vi "Status Page.vi"(8 "Error in":errorcluster, 11 "INL DNL Test in":refnum<class "INL DNL Test.lvclass">) -> (0 "Error out":errorcluster, 3 "INL DNL Test out":refnum<class "INL DNL Test.lvclass">)   [LabVIEW 2020, in "INL DNL Test.lvclass"]
doc: "Status page which displays the DNL and INL results in graph. It also plots the transfer function and plot it in XY graph."
uses:
  INL DNL Test.lvclass
  D:/SDLC/Class/INL DNL Test/Test/Parent/Test.lvclass
  Typedef/User event controls.ctl
  Typedef/Queue Operation.ctl
  Class/INL DNL Test/Device/Parent/Typedef/Data Cluster.ctl
  Class/INL DNL Test/Device/Parent/Device.lvclass
  INL DNL Test.lvclass/INL DNL Test.ctl
  DNL INL Test.lvlib
panel:
  in  "Tab Control":enum32{"Status and graph", "Transfer Function"}(tab)
  out "INL Plot":cluster{"X Values":dbl[], "Y Values":dbl[]}(graph)
  out "DNL Plot":T1(graph)
  in  "Show Tranfer Function":bool
  out "INL":dbl
  out "DNL":dbl
  out "Code":i32
  out "Transfer Function":T2(graph)
  in  "Show DNL INL graph":bool
  # "Note:\nClick run test button to calculate and plot results in graph"
  # "Status and Graph"
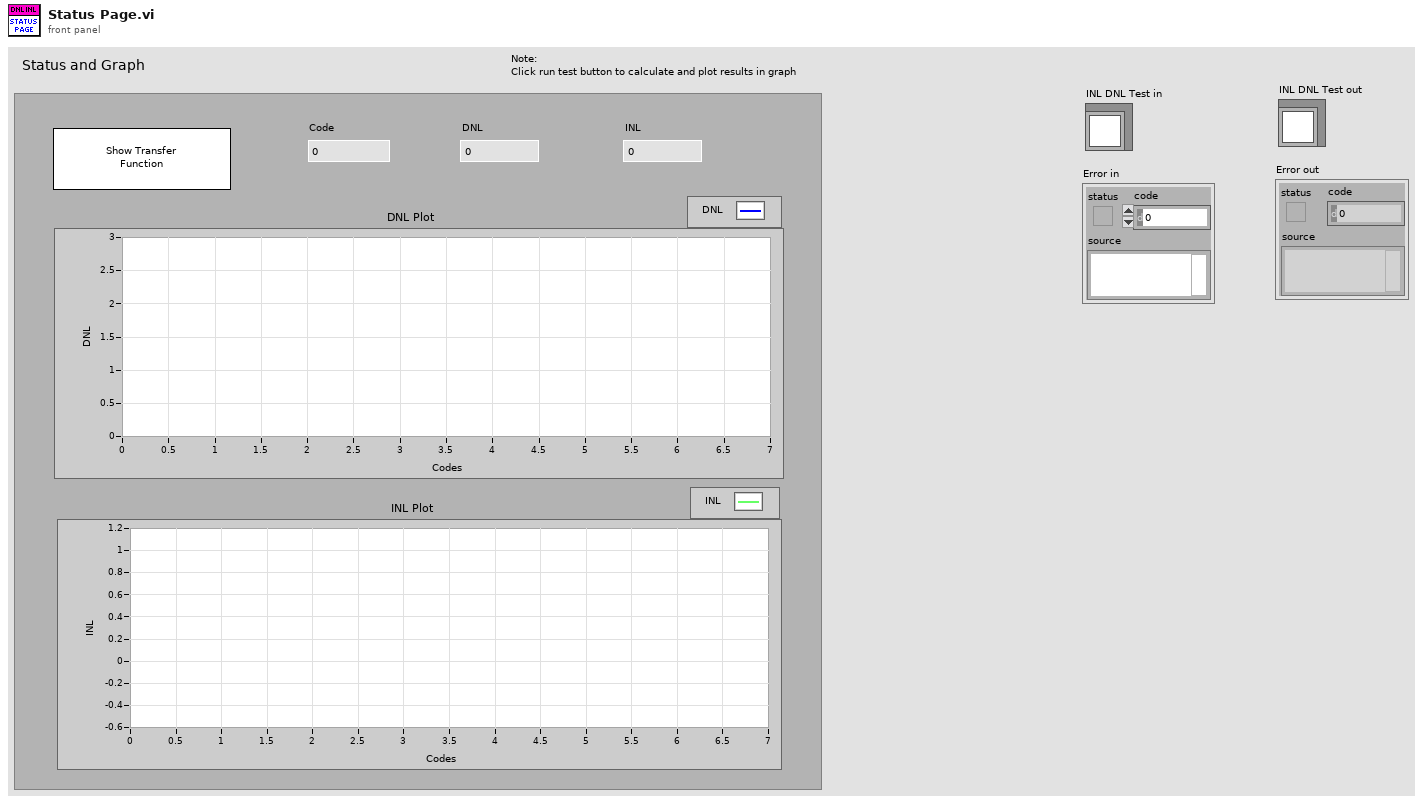
[diagram p1: front panel]
types:
  T1 = cluster{"Ideal Values":dbl[], "Deviated Values":dbl[]}
  T2 = cluster{"Ideal Vlaues":dbl[], "Deviated Values":dbl[]}[]
  T3 = typedef "DNL INL Test.lvlib/Queue Operation.ctl" = enum16{"Create Queue", "Enqueue", "Dequeue", "Enstack", "Flush Queue", "Release Queue"}
  T4 = typedef "DNL INL Test.lvlib/User event controls.ctl" = enum16{"Create", "Generate", "Run Test", "Get Ref", "Destroy"}
  T5 = typedef "Device.lvclass/Data Cluster.ctl" = cluster{"X Values":dbl[], "Y Values":dbl[]}
  T6 = typedef "LVPoint32TypeDef.ctl" = cluster{"Horizontal":i32, "Vertical":i32}
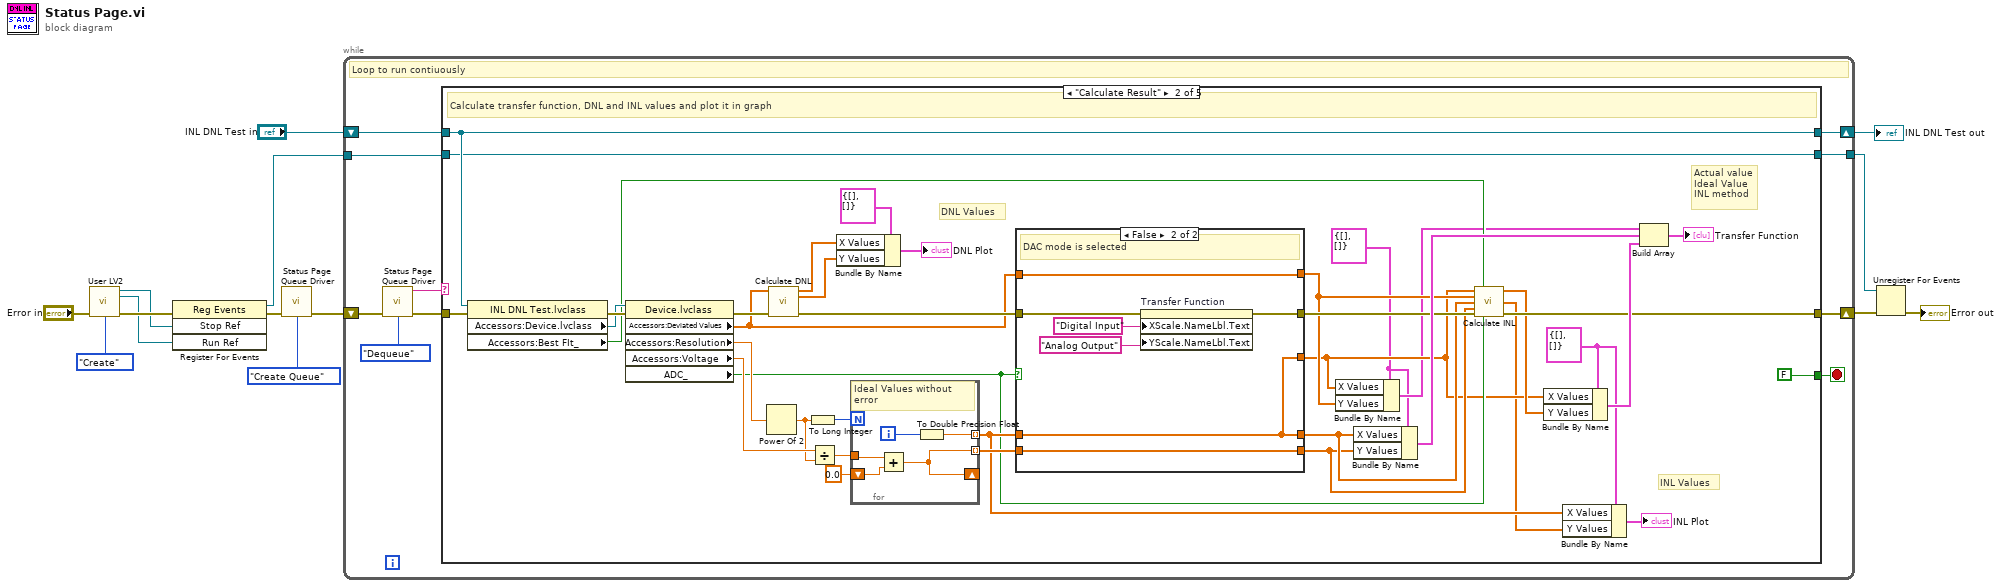
[diagram p0: block diagram]
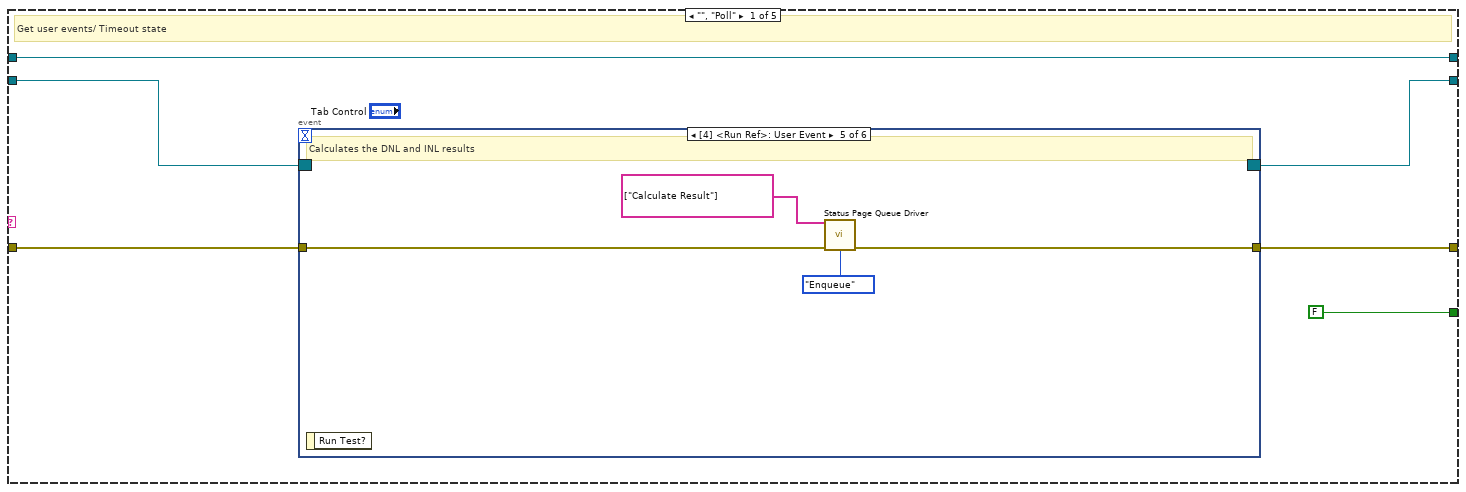
[diagram p2: hidden frame]
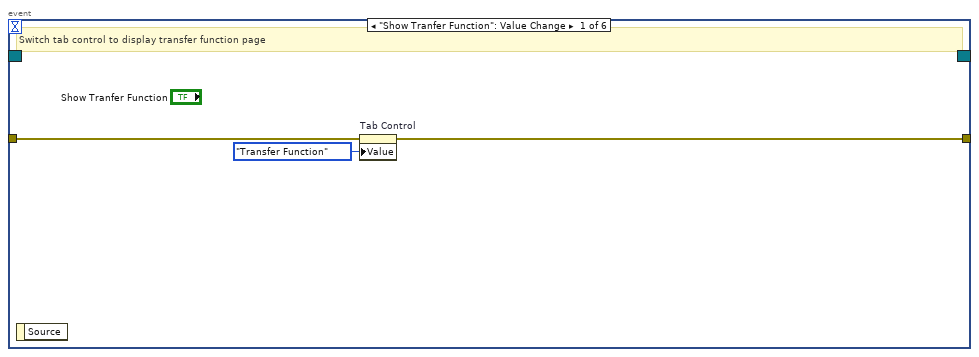
[diagram p3: hidden frame]
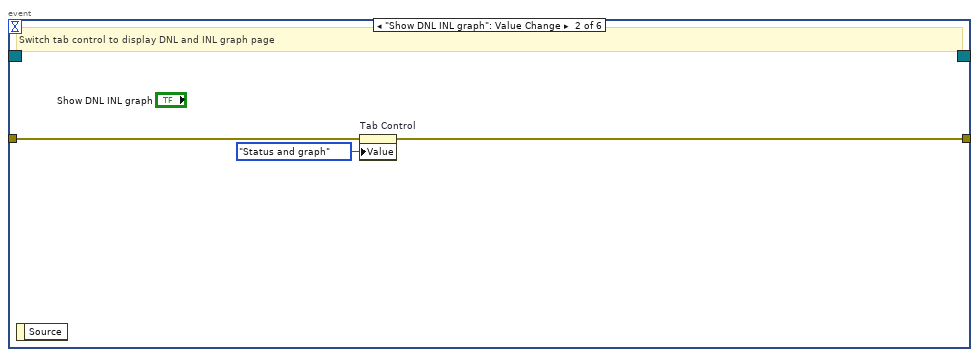
[diagram p4: hidden frame]
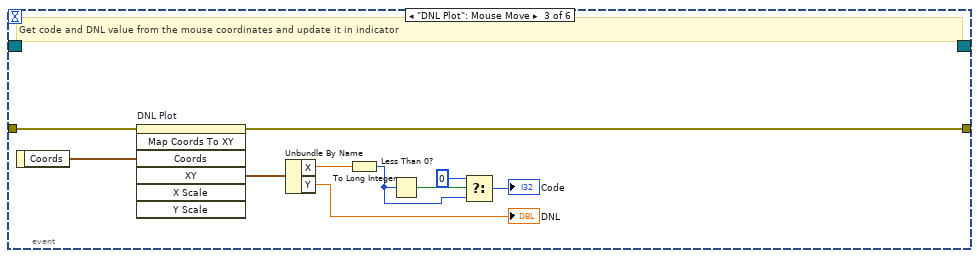
[diagram p5: hidden frame]
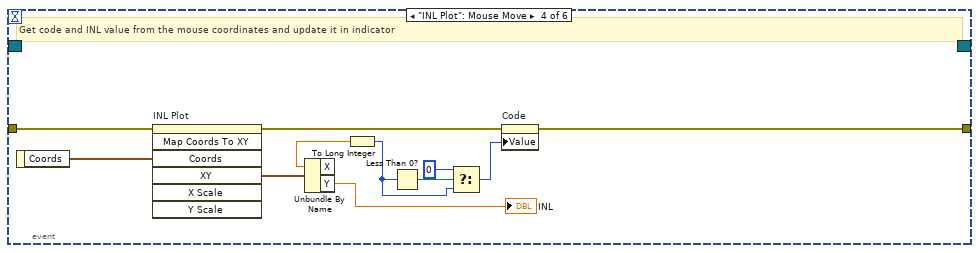
[diagram p6: hidden frame]
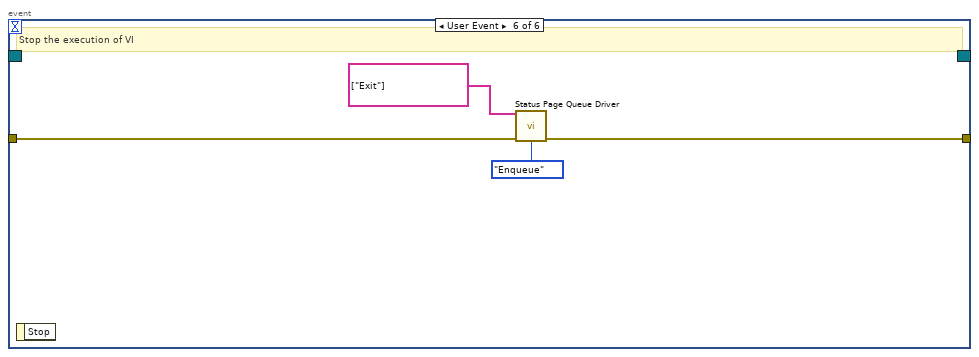
[diagram p7: hidden frame]
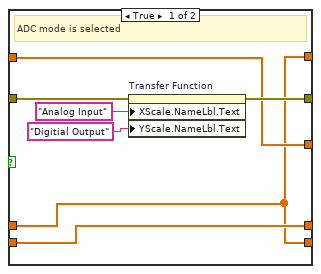
[diagram p8: hidden frame]
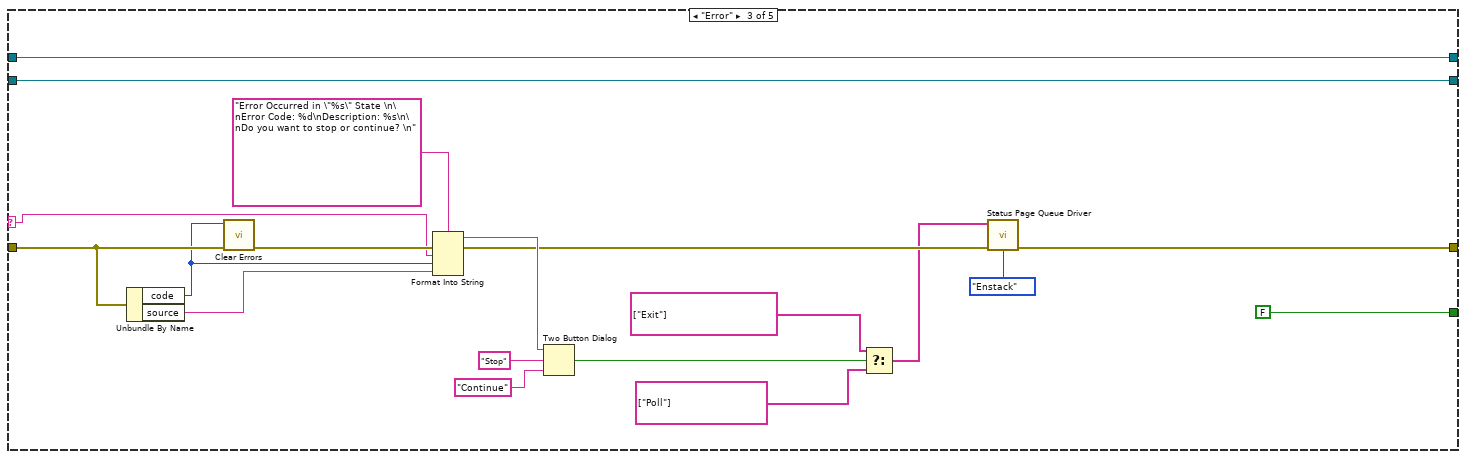
[diagram p9: hidden frame]
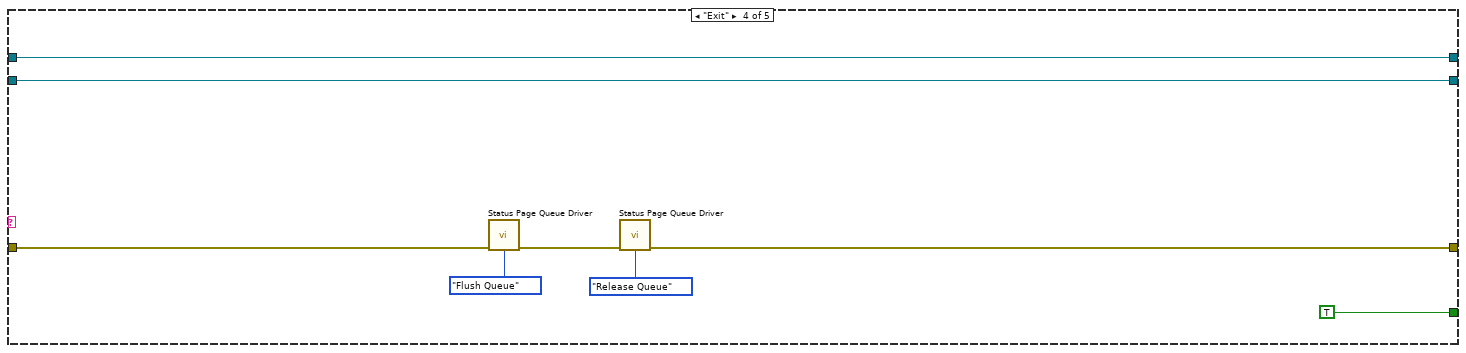
[diagram p10: hidden frame]
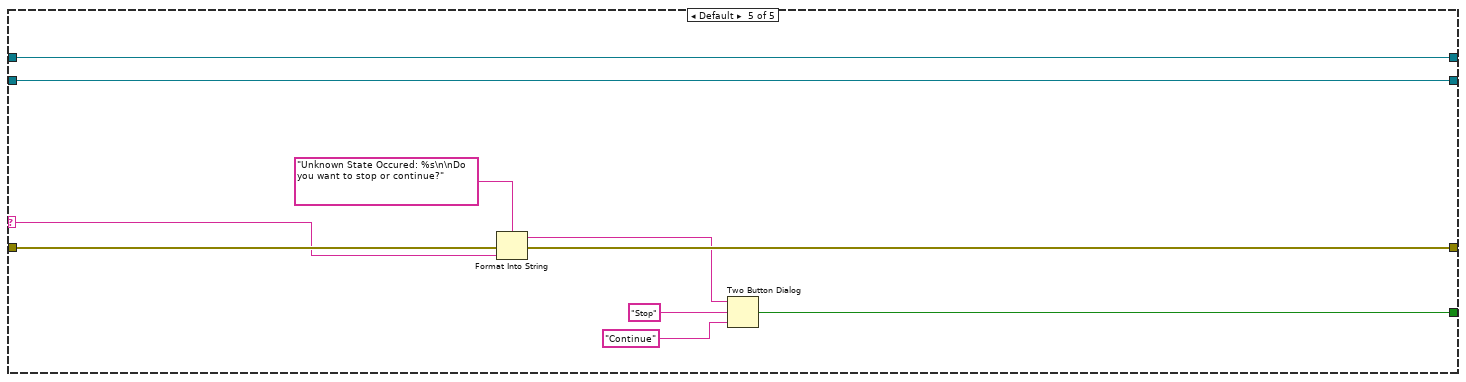
[diagram p11: hidden frame]
diagram:
  n1 = call "User LV2.vi"("Error In"="Error in", "User event controls"=User_event_controls."Create") -> ("Stop Ref"=w11:refnum<user-event>, "Run Ref"=w4:refnum<user-event>, "Error Out"=w12:errorcluster)  [unwired: 11 in]
  n2 = register-events(error in=w12, w11, w4) -> (reference out=w10:refnum<event-registration>, error out=w3:errorcluster)  [unwired: 1 in]
  n3 = call "Status Page Queue Driver.vi"("Error in"=w3, "Queue Operation"=Queue_Operation."Create Queue") -> ("Error out"=w1:errorcluster)  [unwired: 12 in, 1 out]
  n4 = while {
    shift-right: [w24] -> w9
    shift-left: w1 -> [w16]
    tunnel: w10 -> [w23]
    tunnel: [w21] -> w7
    shift-right: [w19] -> w5
    shift-left: "INL DNL Test in" -> [w20]
    stop <- w22 stop-if-true
    # "Loop to run contiuously"
    n5 = call "Status Page Queue Driver.vi"("Error in"=w16, "Queue Operation"=Queue_Operation."Dequeue") -> ("Dequeue Element"=w15:string, "Error out"=w17:errorcluster)  [unwired: 12 in]
    n6 = case shown="\"Calculate Result\"" w15 {
      selector: w15 -> [_ _ w136 _ w154]
      tunnel: w17 -> [w30 w94 w138 w147 w159]
      tunnel: [w29 w76 w128 w143 w156] -> w24
      tunnel: w23 -> [w28 w91 w141 w149 w158]
      tunnel: [FALSE ("Stop") FALSE ("Stop") FALSE ("T button?") TRUE ("Stop") w150] -> w22
      tunnel: [w27 w91 w141 w149 w158] -> w21
      tunnel: w20 -> [w25 w93 w140 w148 w157]
      tunnel: [w25 w93 w140 w148 w157] -> w19
      frame "", "Poll" {
        # "Get user events/ Timeout state"
        n7 = event shown="[4] <Run Ref>: User Event" {
          selector: w28 -> [_ _ _ _ _ _]
          dyn-events: [_ _ _ _ _ _] -> w27
          timeout: _ -> [_ _ _ _ _ _]
          tunnel: w30 -> [w33 w36 w46 w57 w61 w65]
          tunnel: [w32 w35 w45 w52 w60 w64] -> w29
          event "Show Tranfer Function": Value Change {
            # "Switch tab control to display transfer function page"
            n8 = event-data() -> ()  [unwired: 1 in, 1 out]
            n9 = property on="Tab Control" class="TabCtl (strict)"(error in=w33, "Value"=enum32{"Status and graph", "Transfer Function"}."Transfer Function" ("Tab Control")) -> (error out=w32:errorcluster)  [unwired: 1 in, 1 out]
          }
          event "Show DNL INL graph": Value Change {
            # "Switch tab control to display DNL and INL graph page"
            n10 = event-data() -> ()  [unwired: 1 in, 1 out]
            n11 = property on="Tab Control" class="TabCtl (strict)"(error in=w36, "Value"=enum32{"Status and graph", "Transfer Function"}."Status and graph" ("Tab Control")) -> (error out=w35:errorcluster)  [unwired: 1 in, 1 out]
          }
          event "DNL Plot": Mouse Move {
            # "Get code and DNL value from the mouse coordinates and update it in indicator"
            n12 = event-data() -> ("Coords"=w44:T6)  [unwired: 1 in]
            n13 = invoke on="DNL Plot" class="XYGraph (strict)" method="Map Coords To XY"(error in=w46, "Coords"=w44) -> (error out=w45:errorcluster, "XY"=w43:cluster{"X":dbl, "Y":dbl})  [unwired: 5 in, 5 out]
            n14 = Unbundle By Name(w43) -> ("X"=w42:dbl, "Y"=→"DNL":dbl)
            n15 = To Long Integer(number=w42) -> (32bit integer=w39:i32)
            n16 = Less Than 0?(x=w39) -> (x < 0?=w40:bool)
            n17 = Select(t=0, s=w40, f=w39) -> (s? t:f=→"Code":i32)
          }
          event "INL Plot": Mouse Move {
            # "Get code and INL value from the mouse coordinates and update it in indicator"
            n18 = event-data() -> ("Coords"=w55:T6)  [unwired: 1 in]
            n19 = invoke on="INL Plot" class="XYGraph (strict)" method="Map Coords To XY"(error in=w57, "Coords"=w55) -> (error out=w56:errorcluster, "XY"=w54:cluster{"X":dbl, "Y":dbl})  [unwired: 5 in, 5 out]
            n20 = Unbundle By Name(w54) -> ("X"=w51:dbl, "Y"=→"INL":dbl)
            n21 = To Long Integer(number=w51) -> (32bit integer=w49:i32)
            n22 = Less Than 0?(x=w49) -> (x < 0?=w50:bool)
            n23 = Select(t=0, s=w50, f=w49) -> (s? t:f=w47:i32)
            n24 = property on="Code" class="DigNum (strict)"(error in=w56, "Value"=w47) -> (error out=w52:errorcluster)  [unwired: 1 in, 1 out]
          }
          event User Event {
            # "Calculates the DNL and INL results"
            n25 = event-data() -> ()  [unwired: 1 in, 1 out]
            n26 = call "Status Page Queue Driver.vi"("States"=string[] ["Calculate Result"], "Error in"=w61, "Queue Operation"=Queue_Operation."Enqueue") -> ("Error out"=w60:errorcluster)  [unwired: 11 in, 1 out]
          }
          event User Event {
            # "Stop the execution of VI"
            n27 = event-data() -> ()  [unwired: 1 in, 1 out]
            n28 = call "Status Page Queue Driver.vi"("States"=string[] ["Exit"], "Error in"=w65, "Queue Operation"=Queue_Operation."Enqueue") -> ("Error out"=w64:errorcluster)  [unwired: 11 in, 1 out]
          }
        }
      }
      frame "Calculate Result" {
        w66 = T5 {"X Values"=[], "Y Values"=[]} ("Cluster")
        w88 = T5 {"X Values"=[], "Y Values"=[]} ("Cluster")
        # "INL Values"
        # "Actual value\nIdeal Value\nINL method"
        # "DNL Values"
        # "Calculate transfer function, DNL and INL values and plot it in graph"
        n29 = property class="INL DNL Test.lvclass"(reference=w93, error in=w94) -> (error out=w103:errorcluster, "Accessors:Device.lvclass"=w102:refnum<class "Device.lvclass">, "Accessors:Best FIt_"=w72:bool)  [unwired: 1 out]
        n30 = property class="Device.lvclass"(reference=w102, error in=w103) -> (error out=w84:errorcluster, "Accessors:Deviated Values"=w79:dbl[], "Accessors:Resolution"=w101:dbl, "Accessors:Voltage"=w99:dbl, "ADC_"=w71:bool)  [unwired: 1 out]
        n31 = Power Of 2(x=w101) -> (2^x=w80:dbl)
        n32 = call "Calculate DNL.vi"("Deviated Values"=w79, "Error in"=w84) -> ("Codes"=w82:dbl[], "DNL Values"=w81:dbl[], "Error out"=w83:errorcluster)  [unwired: 11 in]
        n33 = To Long Integer(number=w80) -> (32bit integer=w100:i32)
        n34 = Divide(x=w99, y=w80) -> (x/y=w98:dbl)
        n35 = Bundle By Name(cluster=T5 {"X Values"=[], "Y Values"=[]} ("Cluster"), "X Values"=w82, "Y Values"=w81) -> (→"DNL Plot":T5)
        n36 = for {
          N: w100 -> [_]
          tunnel: w98 -> [w108]
          shift-right: [w106] -> _
          shift-left: 0.0 ("y") -> [w107]
          tunnel: [w106] -> w85 mode=indexing
          tunnel: [w104] -> w78 mode=indexing
          i -> [w105]
          # "Ideal Values without error"
          n37 = Add(x=w108, y=w107) -> (x+y=w106:dbl)
          n38 = To Double Precision Float(number=w105) -> (double precision float=w104:dbl)
        }
        n39 = case shown="False" w71 {
          tunnel: w83 -> [w115 w122]
          tunnel: w78 -> [w109 w118]
          tunnel: w85 -> [w111 w116]
          tunnel: [w114 w121] -> w77
          tunnel: [w111 w118] -> w74
          tunnel: [w109 w116] -> w73
          tunnel: w79 -> [w110 w117]
          tunnel: [w109 w117] -> w75
          tunnel: [w110 w118] -> w69
          frame True {
            # "ADC mode is selected"
            n40 = property on="Transfer Function" class="XYGraph (strict)"(error in=w115, "XScale.NameLbl.Text"="Analog Input" ("X Scale.Name Label.Text"), "YScale.NameLbl.Text"="Digitial Output" ("Y Scale.Name Label.Text")) -> (error out=w114:errorcluster)  [unwired: 1 in, 1 out]
          }
          frame False {
            # "DAC mode is selected"
            n41 = property on="Transfer Function" class="XYGraph (strict)"(error in=w122, "XScale.NameLbl.Text"="Digital Input" ("X Scale.Name Label.Text"), "YScale.NameLbl.Text"="Analog Output" ("Y Scale.Name Label.Text")) -> (error out=w121:errorcluster)  [unwired: 1 in, 1 out]
          }
        }
        n42 = Bundle By Name(cluster=w66, "X Values"=w69, "Y Values"=w75) -> (w67:T5)
        n43 = Bundle By Name(cluster=w66, "X Values"=w74, "Y Values"=w73) -> (w95:T5)
        n44 = call "Calculate INL.vi"("Actual X"=w69, "Best Fit?"=w72, "Actual Y"=w75, "Ideal X"=w74, "Ideal Y"=w73, "Error in"=w77, "ADC?"=w71) -> ("INL Y Plot Values"=w70:dbl[], "INL Result values"=w68:dbl[], "Error out"=w76:errorcluster)  [unwired: 6 in]
        n45 = Bundle By Name(cluster=w88, "X Values"=w69, "Y Values"=w70) -> (w96:T5)
        n46 = Bundle By Name(cluster=w88, "X Values"=w78, "Y Values"=w68) -> (→"INL Plot":T5)
        n47 = Build Array(w67, w95, w96) -> (→"Transfer Function":T5[])
      }
      frame "Error" {
        n48 = Unbundle By Name(w138) -> ("code"=w135:i32, "source"=w134:string)
        n49 = call <vilib>:"Clear Errors.vi"("error in (no error)"=w138, "specific error code to clear (0: all)"=w135) -> ("error out"=w137:errorcluster)  [unwired: 4 in, 1 out]
        n50 = Format Into String(format string="Error Occurred in \"%s\" State \n\nError Code: %d\nDescription: %s\n\nDo you want to stop or continue? \n", error in=w137, w136, w135, w134) -> (resulting string=w133:string, error out=w129:errorcluster)  [unwired: 1 in]
        n51 = Two Button Dialog(message=w133, 1:"Continue" ("F button name (\"Cancel\")"), 2:"Stop" ("T button name (\"OK\")")) -> (T button?=w130:bool)
        n52 = Select(t=string[] ["Exit"] ("States"), s=w130, f=string[] ["Poll"]) -> (s? t:f=w125:string[])
        n53 = call "Status Page Queue Driver.vi"("States"=w125, "Error in"=w129, "Queue Operation"=Queue_Operation."Enstack") -> ("Error out"=w128:errorcluster)  [unwired: 11 in, 1 out]
      }
      frame "Exit" {
        n54 = call "Status Page Queue Driver.vi"("Error in"=w147, "Queue Operation"=Queue_Operation."Flush Queue") -> ("Error out"=w145:errorcluster)  [unwired: 12 in, 1 out]
        n55 = call "Status Page Queue Driver.vi"("Error in"=w145, "Queue Operation"=Queue_Operation."Release Queue") -> ("Error out"=w143:errorcluster)  [unwired: 12 in, 1 out]
      }
      frame Default {
        n56 = Format Into String(format string="Unknown State Occured: %s\n\nDo you want to stop or continue?", error in=w159, w154) -> (resulting string=w153:string, error out=w156:errorcluster)  [unwired: 1 in]
        n57 = Two Button Dialog(message=w153, 1:"Continue" ("F button name (\"Cancel\")"), 2:"Stop" ("T button name (\"OK\")")) -> (T button?=w150:bool)
      }
    }
  }
  "INL DNL Test out" <- w5
  n58 = Unregister For Events(event registration refnum=w7, error in=w9) -> (error out=→"Error out":errorcluster)
